vi "Introduce.vi"(8 "Error In":errorcluster, 11 "Astromech droid In":refnum<class "Astromech droid.lvclass">) -> (0 "Error Out":errorcluster, 3 "Astromech droid Out":refnum<class "Astromech droid.lvclass">)   [LabVIEW 2021, in "Astromech droid.lvclass"]
doc: "Show ID of droid in prompt message for user. Comments in Polish."
uses:
  Astromech droid.lvclass
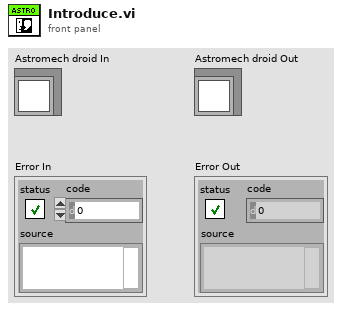
[diagram p1: front panel]
types:
  T1 = enum16{"Q-Series", "BB-Series", "C-Series", "R-Series"}
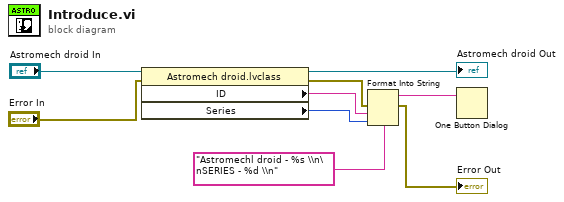
[diagram p0: block diagram]
diagram:
  n1 = property class="Astromech droid.lvclass"(reference="Astromech droid In", error in="Error In") -> (reference out=→"Astromech droid Out":refnum<class "Astromech droid.lvclass">, error out=w4:errorcluster, "ID"=w7:string, "Series"=w6:T1)
  n2 = Format Into String(format string="Astromechl droid - %s \\n\nSERIES - %d \\n", error in=w4, w7, w6) -> (resulting string=w1:string, error out=→"Error Out":errorcluster)  [unwired: 1 in]
  n3 = One Button Dialog(message=w1) -> ()  [unwired: 1 in, 1 out]
